vi "Get Desired Size.vi"(8 "error in (no error)":errorcluster, 11 "2DArrayPanel in":refnum<class "2DArrayPanel.lvclass">) -> (0 "error out":errorcluster, 2 "Desired Size":T1, 3 "2DArrayPanel out":refnum<class "2DArrayPanel.lvclass">)   [LabVIEW 2020, in "2D Array Example.lvlib" / "2DArrayPanel.lvclass"]
uses:
  2DArrayPanel.lvclass
  2DArrayPanel.lvclass/2DArrayPanel.ctl
  OOPanel/ArrayPanel/Desired Size.ctl
  OOPanel/OOPanel.lvlib
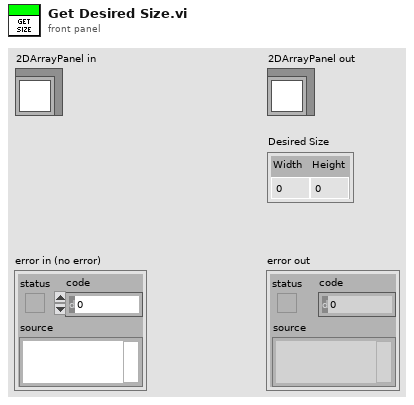
[diagram p1: front panel]
types:
  T1 = typedef "OOPanel.lvlib/Desired Size.ctl" = cluster{"Width":u32, "Height":u32}
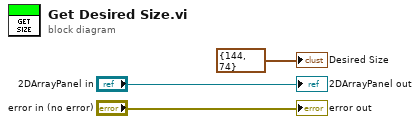
[diagram p0: block diagram]
diagram:
  "error out" <- "error in (no error)"
  "2DArrayPanel out" <- "2DArrayPanel in"
  "Desired Size" <- T1 {"Width"=144, "Height"=74} ("Desired Size")
